vi "数据初始化(子VI).vi"(8 "错误常量 2":errorcluster caption="错误常量", 11 "Array输入":refnum<vi>) -> (0 "错误常量":errorcluster)   [LabVIEW 2016]
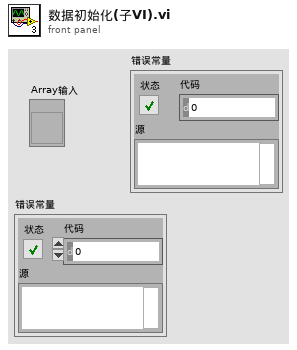
[diagram p1: front panel]
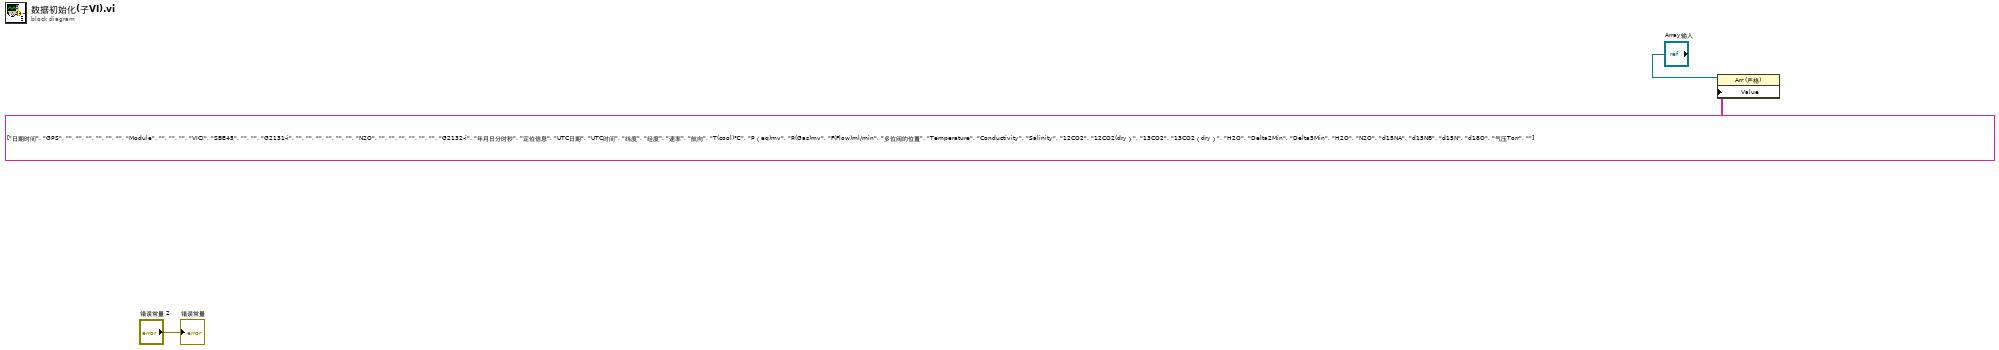
[diagram p0: block diagram]
diagram:
  n1 = property class="Arr (严格)"(reference="Array输入", "Value"=string[][] [["日期时间", "GPS", "", "", "", "", "", "", "Module", "", "", "", "VICI", "SBE45", "", "", "G2131-i", "", "", "", "", "", "", "N2O", "", "", "", "", "", "", "G2132-i"], ["年月日分时秒", "定位信息", "UTC日期", "UTC时间", "纬度", "经度", "速率", "航向", "T(cool)℃", "P（eq)mv", "R(Gas)mv", "F(Flow)ml/min", "多位阀的位置", "Temperature", "Conductivity", "Salinity", "12CO2", "12CO2(dry）", "13CO2", "13CO2（dry）", "H2O", "Delta2Min", "Delta5Min", "H2O", "N2O", "d15NA", "d15NB", "d15N", "d18O", "气压Torr", ""]] ("数据数组")) -> ()  [unwired: 1 in, 2 out]
  "错误常量" <- "错误常量 2"
